vi "Create Serial Output Channel CSI-2 IO x4.vi"() -> (4 "serial output channel csi-2 io x4 2":T4)   [LabVIEW 2020, in "GettingStarted_Common_148X_FPGA.lvlib"]
uses:
  GettingStarted_Common_148X_FPGA.lvlib
  Types/Serial Output Channel IO.ctl
  Types/Serial Output Channel IO 32b.ctl
  Types/Serial Output Channel IO 64b.ctl
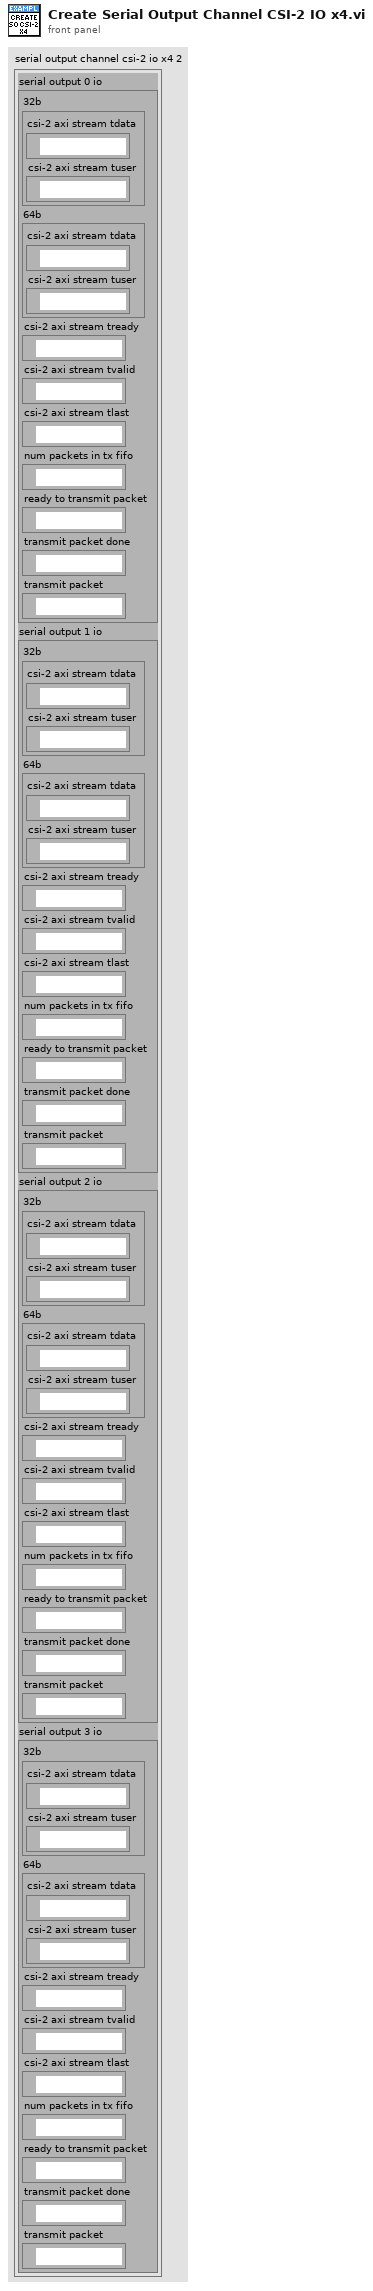
[diagram p1: front panel]
types:
  T1 = typedef "GettingStarted_Common_148X_FPGA.lvlib/Serial Output Channel IO.ctl" = cluster{"32b":T2, "64b":T3, "csi-2 axi stream tready":refnum<k21>, "csi-2 axi stream tvalid":refnum<k21>, "csi-2 axi stream tlast":refnum<k21>, "num packets in tx fifo":refnum<k21>, "ready to transmit packet":refnum<k21>, "transmit packet done":refnum<k21>, "transmit packet":refnum<k21>}
  T2 = typedef "GettingStarted_Common_148X_FPGA.lvlib/Serial Output Channel IO 32b.ctl" = cluster{"csi-2 axi stream tdata":refnum<k21>, "csi-2 axi stream tuser":refnum<k21>}
  T3 = typedef "GettingStarted_Common_148X_FPGA.lvlib/Serial Output Channel IO 64b.ctl" = cluster{"csi-2 axi stream tdata":refnum<k21>, "csi-2 axi stream tuser":refnum<k21>}
  T4 = cluster{"serial output 0 io":T1, "serial output 1 io":T1, "serial output 2 io":T1, "serial output 3 io":T1}
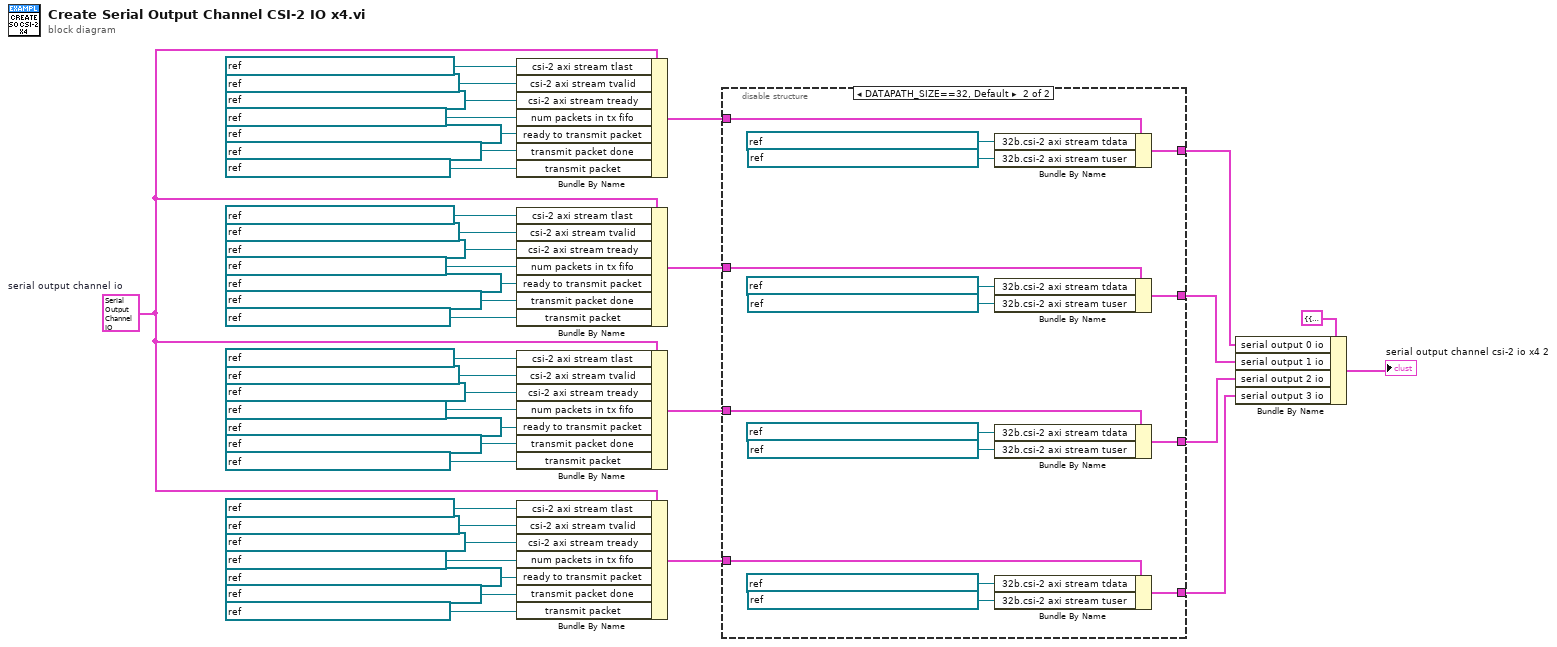
[diagram p0: block diagram]
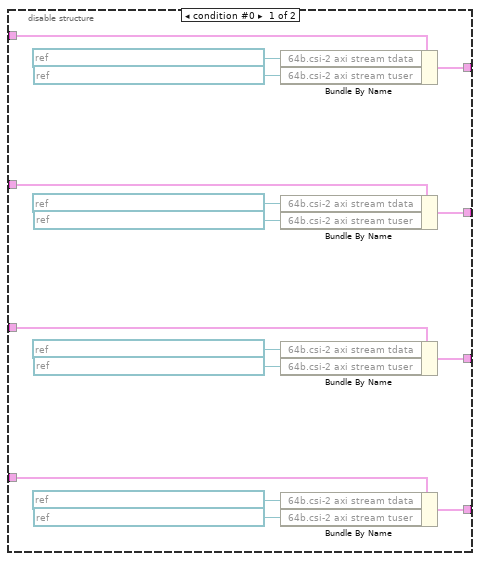
[diagram p2: hidden frame]
diagram:
  w14 = T1 {"32b"={"csi-2 axi stream tdata"="", "csi-2 axi stream tuser"=""}, "64b"={"csi-2 axi stream tdata"="", "csi-2 axi stream tuser"=""}, "csi-2 axi stream tready"="", "csi-2 axi stream tvalid"="", "csi-2 axi stream tlast"="", "num packets in tx fifo"="", "ready to transmit packet"="", "transmit packet done"="", "transmit packet"=""}  # serial output channel io
  n1 = Bundle By Name(cluster=w14, "csi-2 axi stream tlast"=refnum<k21> "IO Socket\\SO 0 CSI-2 AXI Stream TLast", "csi-2 axi stream tvalid"=refnum<k21> "IO Socket\\SO 0 CSI-2 AXI Stream TValid", "csi-2 axi stream tready"=refnum<k21> "IO Socket\\SO 0 CSI-2 AXI Stream TReady", "num packets in tx fifo"=refnum<k21> "IO Socket\\SO 0 CSI-2 Packets In FIFO", "ready to transmit packet"=refnum<k21> "IO Socket\\SO 0 CSI-2 Ready To Transmit Packet", "transmit packet done"=refnum<k21> "IO Socket\\SO 0 CSI-2 Transmit Packet Done", "transmit packet"=refnum<k21> "IO Socket\\SO 0 CSI-2 Transmit Packet") -> (w8:T1)
  n2 = Bundle By Name(cluster=w14, "csi-2 axi stream tlast"=refnum<k21> "IO Socket\\SO 1 CSI-2 AXI Stream TLast", "csi-2 axi stream tvalid"=refnum<k21> "IO Socket\\SO 1 CSI-2 AXI Stream TValid", "csi-2 axi stream tready"=refnum<k21> "IO Socket\\SO 1 CSI-2 AXI Stream TReady", "num packets in tx fifo"=refnum<k21> "IO Socket\\SO 1 CSI-2 Packets In FIFO", "ready to transmit packet"=refnum<k21> "IO Socket\\SO 1 CSI-2 Ready To Transmit Packet", "transmit packet done"=refnum<k21> "IO Socket\\SO 1 CSI-2 Transmit Packet Done", "transmit packet"=refnum<k21> "IO Socket\\SO 1 CSI-2 Transmit Packet") -> (w7:T1)
  n3 = Bundle By Name(cluster=w14, "csi-2 axi stream tlast"=refnum<k21> "IO Socket\\SO 2 CSI-2 AXI Stream TLast", "csi-2 axi stream tvalid"=refnum<k21> "IO Socket\\SO 2 CSI-2 AXI Stream TValid", "csi-2 axi stream tready"=refnum<k21> "IO Socket\\SO 2 CSI-2 AXI Stream TReady", "num packets in tx fifo"=refnum<k21> "IO Socket\\SO 2 CSI-2 Packets In FIFO", "ready to transmit packet"=refnum<k21> "IO Socket\\SO 2 CSI-2 Ready To Transmit Packet", "transmit packet done"=refnum<k21> "IO Socket\\SO 2 CSI-2 Transmit Packet Done", "transmit packet"=refnum<k21> "IO Socket\\SO 2 CSI-2 Transmit Packet") -> (w6:T1)
  n4 = Bundle By Name(cluster=w14, "csi-2 axi stream tlast"=refnum<k21> "IO Socket\\SO 3 CSI-2 AXI Stream TLast", "csi-2 axi stream tvalid"=refnum<k21> "IO Socket\\SO 3 CSI-2 AXI Stream TValid", "csi-2 axi stream tready"=refnum<k21> "IO Socket\\SO 3 CSI-2 AXI Stream TReady", "num packets in tx fifo"=refnum<k21> "IO Socket\\SO 3 CSI-2 Packets In FIFO", "ready to transmit packet"=refnum<k21> "IO Socket\\SO 3 CSI-2 Ready To Transmit Packet", "transmit packet done"=refnum<k21> "IO Socket\\SO 3 CSI-2 Transmit Packet Done", "transmit packet"=refnum<k21> "IO Socket\\SO 3 CSI-2 Transmit Packet") -> (w5:T1)
  n5 = disable-structure shown="DATAPATH_SIZE==32, Default" {
    disable-tunnel: [w41 w65] -> w4
    disable-tunnel: [w40 w64] -> w1
    disable-tunnel: [w43 w67] -> w2
    disable-tunnel: [w42 w66] -> w3
    disable-tunnel: w8 -> [w51 w71]
    disable-tunnel: w7 -> [w50 w70]
    disable-tunnel: w6 -> [w49 w69]
    disable-tunnel: w5 -> [w48 w68]
    frame condition #0 {
      n6 = Bundle By Name(cluster=w51, "64b.csi-2 axi stream tdata"=refnum<k21> "IO Socket\\SO 0 CSI-2 AXI Stream TData" ("csi-2 axi stream tdata"), "64b.csi-2 axi stream tuser"=refnum<k21> "IO Socket\\SO 0 CSI-2 AXI Stream TUser" ("csi-2 axi stream tuser")) -> (w40:T1)
      n7 = Bundle By Name(cluster=w50, "64b.csi-2 axi stream tdata"=refnum<k21> "IO Socket\\SO 1 CSI-2 AXI Stream TData" ("csi-2 axi stream tdata"), "64b.csi-2 axi stream tuser"=refnum<k21> "IO Socket\\SO 1 CSI-2 AXI Stream TUser" ("csi-2 axi stream tuser")) -> (w43:T1)
      n8 = Bundle By Name(cluster=w49, "64b.csi-2 axi stream tdata"=refnum<k21> "IO Socket\\SO 2 CSI-2 AXI Stream TData" ("csi-2 axi stream tdata"), "64b.csi-2 axi stream tuser"=refnum<k21> "IO Socket\\SO 2 CSI-2 AXI Stream TUser" ("csi-2 axi stream tuser")) -> (w42:T1)
      n9 = Bundle By Name(cluster=w48, "64b.csi-2 axi stream tdata"=refnum<k21> "IO Socket\\SO 3 CSI-2 AXI Stream TData" ("csi-2 axi stream tdata"), "64b.csi-2 axi stream tuser"=refnum<k21> "IO Socket\\SO 3 CSI-2 AXI Stream TUser" ("csi-2 axi stream tuser")) -> (w41:T1)
    }
    frame condition #1 (active) {
      n10 = Bundle By Name(cluster=w71, "32b.csi-2 axi stream tdata"=refnum<k21> "IO Socket\\SO 0 CSI-2 AXI Stream TData" ("csi-2 axi stream tdata"), "32b.csi-2 axi stream tuser"=refnum<k21> "IO Socket\\SO 0 CSI-2 AXI Stream TUser" ("csi-2 axi stream tuser")) -> (w64:T1)
      n11 = Bundle By Name(cluster=w70, "32b.csi-2 axi stream tdata"=refnum<k21> "IO Socket\\SO 1 CSI-2 AXI Stream TData" ("csi-2 axi stream tdata"), "32b.csi-2 axi stream tuser"=refnum<k21> "IO Socket\\SO 1 CSI-2 AXI Stream TUser" ("csi-2 axi stream tuser")) -> (w67:T1)
      n12 = Bundle By Name(cluster=w69, "32b.csi-2 axi stream tdata"=refnum<k21> "IO Socket\\SO 2 CSI-2 AXI Stream TData" ("csi-2 axi stream tdata"), "32b.csi-2 axi stream tuser"=refnum<k21> "IO Socket\\SO 2 CSI-2 AXI Stream TUser" ("csi-2 axi stream tuser")) -> (w66:T1)
      n13 = Bundle By Name(cluster=w68, "32b.csi-2 axi stream tdata"=refnum<k21> "IO Socket\\SO 3 CSI-2 AXI Stream TData" ("csi-2 axi stream tdata"), "32b.csi-2 axi stream tuser"=refnum<k21> "IO Socket\\SO 3 CSI-2 AXI Stream TUser" ("csi-2 axi stream tuser")) -> (w65:T1)
    }
  }
  n14 = Bundle By Name(cluster=T4 {"serial output 0 io"={"32b"={"csi-2 axi stream tdata"="", "csi-2 axi stream tuser"=""}, "64b"={"csi-2 axi stream tdata"="", "csi-2 axi stream tuser"=""}, "csi-2 axi stream tready"="", "csi-2 axi stream tvalid"="", "csi-2 axi stream tlast"="", "num packets in tx fifo"="", "ready to transmit packet"="", "transmit packet done"="", "transmit packet"=""}, "serial output 1 io"={"32b"={"csi-2 axi stream tdata"="", "csi-2 axi stream tuser"=""}, "64b"={"csi-2 axi stream tdata"="", "csi-2 axi stream tuser"=""}, "csi-2 axi stream tready"="", "csi-2 axi stream tvalid"="", "csi-2 axi stream tlast"="", "num packets in tx fifo"="", "ready to transmit packet"="", "transmit packet done"="", "transmit packet"=""}, "serial output 2 io"={"32b"={"csi-2 axi stream tdata"="", "csi-2 axi stream tuser"=""}, "64b"={"csi-2 axi stream tdata"="", "csi-2 axi stream tuser"=""}, "csi-2 axi stream tready"="", "csi-2 axi stream tvalid"="", "csi-2 axi stream tlast"="", "num packets in tx fifo"="", "ready to transmit packet"="", "transmit packet done"="", "transmit packet"=""}, "serial output 3 io"={"32b"={"csi-2 axi stream tdata"="", "csi-2 axi stream tuser"=""}, "64b"={"csi-2 axi stream tdata"="", "csi-2 axi stream tuser"=""}, "csi-2 axi stream tready"="", "csi-2 axi stream tvalid"="", "csi-2 axi stream tlast"="", "num packets in tx fifo"="", "ready to transmit packet"="", "transmit packet done"="", "transmit packet"=""}} ("serial output channel io x4"), "serial output 0 io"=w1, "serial output 1 io"=w2, "serial output 2 io"=w3, "serial output 3 io"=w4) -> (→"serial output channel csi-2 io x4 2":T4)
